vi "Sequencer.pub.vi"() -> ()   [LabVIEW 2014]
uses:
  <vilib>/Analysis/NI_AALPro.lvlib
panel:
  out "Counts":u32[](array[numeric])
  out "PMT4":u32[](array[numeric])
  out "PMT3":u32[](array[numeric])
  out "PMT2":u32[](array[numeric])
  out "PMT1":u32[](array[numeric])
  in  "Threshold":dbl=1.0
  out "CompiledSequence":string="#DopplerCooling\r\n0.9 10100000 00000000 00000000\r\n\r\n#Pump\r\n0.3 01000000 00000000 00000000\r\n\r\n#Pulsed\r\n0.2 00100000 00000000 00000000\r\n0.4 00000100 00000000 00000000\r\n0.2 00000000 10000000 00000000\r\n0.2 01000000 00000000 01000000\n"
  out "ChapterNames":string[](array[string])
  out "ChapterPositions":u32[](array[numeric])
  in  "Scan":enum32{"Time"}(tab)
  out "Now (us)":dbl=1.0 format="%.2f"
  in  "Step (us)":dbl=1.0 format="%.2f"
  in  "End (us)":dbl=1.0 format="%.2f"
  in  "Start (us)":dbl=1.0 format="%.2f"
  in  "Time Scan":bool
  in  "Chapter":u16(ring) items=["Zero", "DopplerCooling[0]", "DopplerCooling[1]", "DopplerCooling[2]", "Zero"]
  in  "Once":bool=TRUE
  in  "Sequencer Port":refnum<visa-resource-name>="COM8"
  in  "Send":bool
  out "Durations Backup":dbl[](array[numeric])
  out "Durations":dbl[](array[numeric])
  in  "Period (ns)":dbl=5.0
  out "States":string[](array[string])
  in  "Sequencer":bool
  in  "Edit":enum32{"Sequence"}(tab)
  in  "Sequence":string
  in  "Save":bool
  in  "Chapter (us)":string
  in  "Sequence File":path=path "D:/Data/Sequence/Cooling.seq"
  in  "Repeats":u32=100
  in  "Compile":bool
  in  "Data":bool
  out "Clock":string
  in  "Detect":enum32{"PMT", "TTL"}(tab)
  in  "4":bool
  in  "3":bool
  in  "2":bool
  in  "1":bool=TRUE
  in  "Save":bool
  in  "Count or State":i16(ring) items=["Count", "State"]
  in  "Fit":bool
  out "Peak":u32
  out "?":cluster{dbl[], "Axis":dbl[]}(graph)
  out "?":cluster{"Axis":dbl[], "Histogram":i32[]}(graph)
  in  "Data Chapter":i16(ring) items=["All", "DopplerCooling[2]"]
  out "Average Counts or States":dbl(graph)
  out "Average of Scans":dbl[](graph)
  out "data file":string
  out "History Data":dbl[](array[numeric])
  in  "Sweep":bool
  out "Digital Waveform Graph":digitaldata(graph)
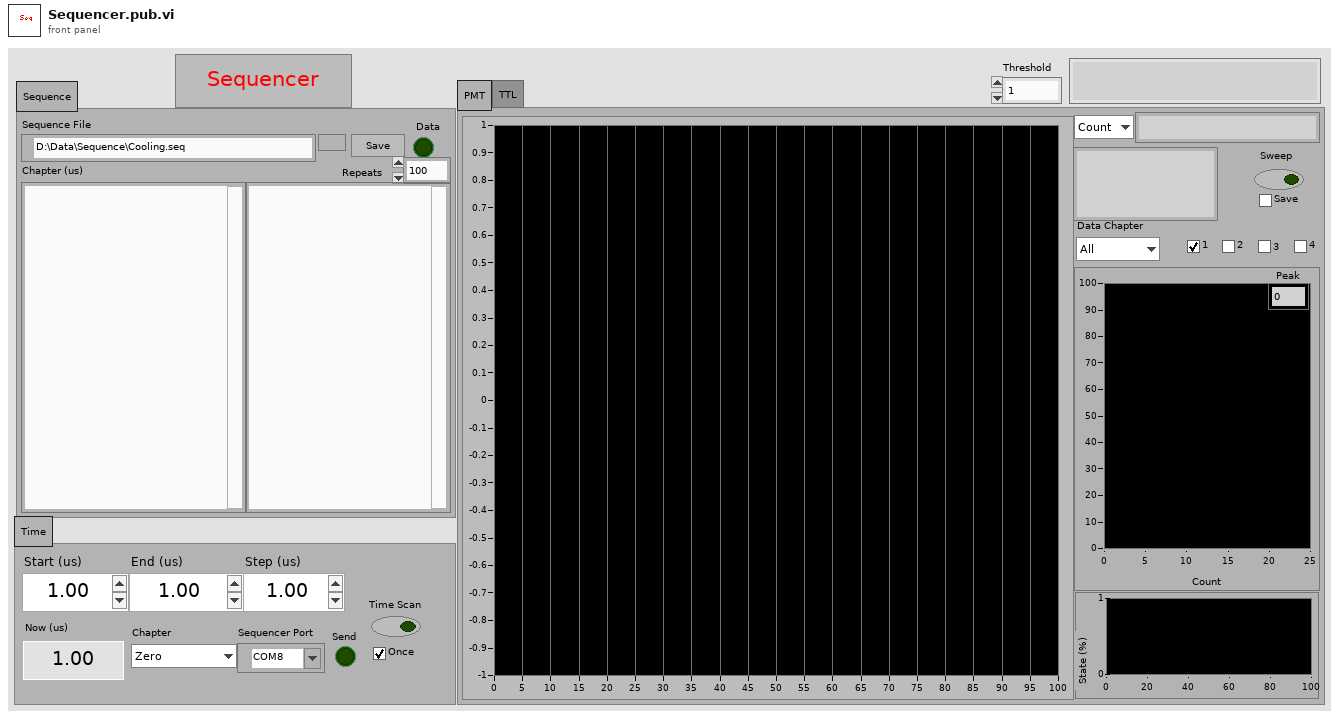
[diagram p1: front panel]
types:
  T1 = cluster{"lower":dbl, "upper":dbl, "inclusion":enum32{"lower", "upper", "both", "neither"}}[]
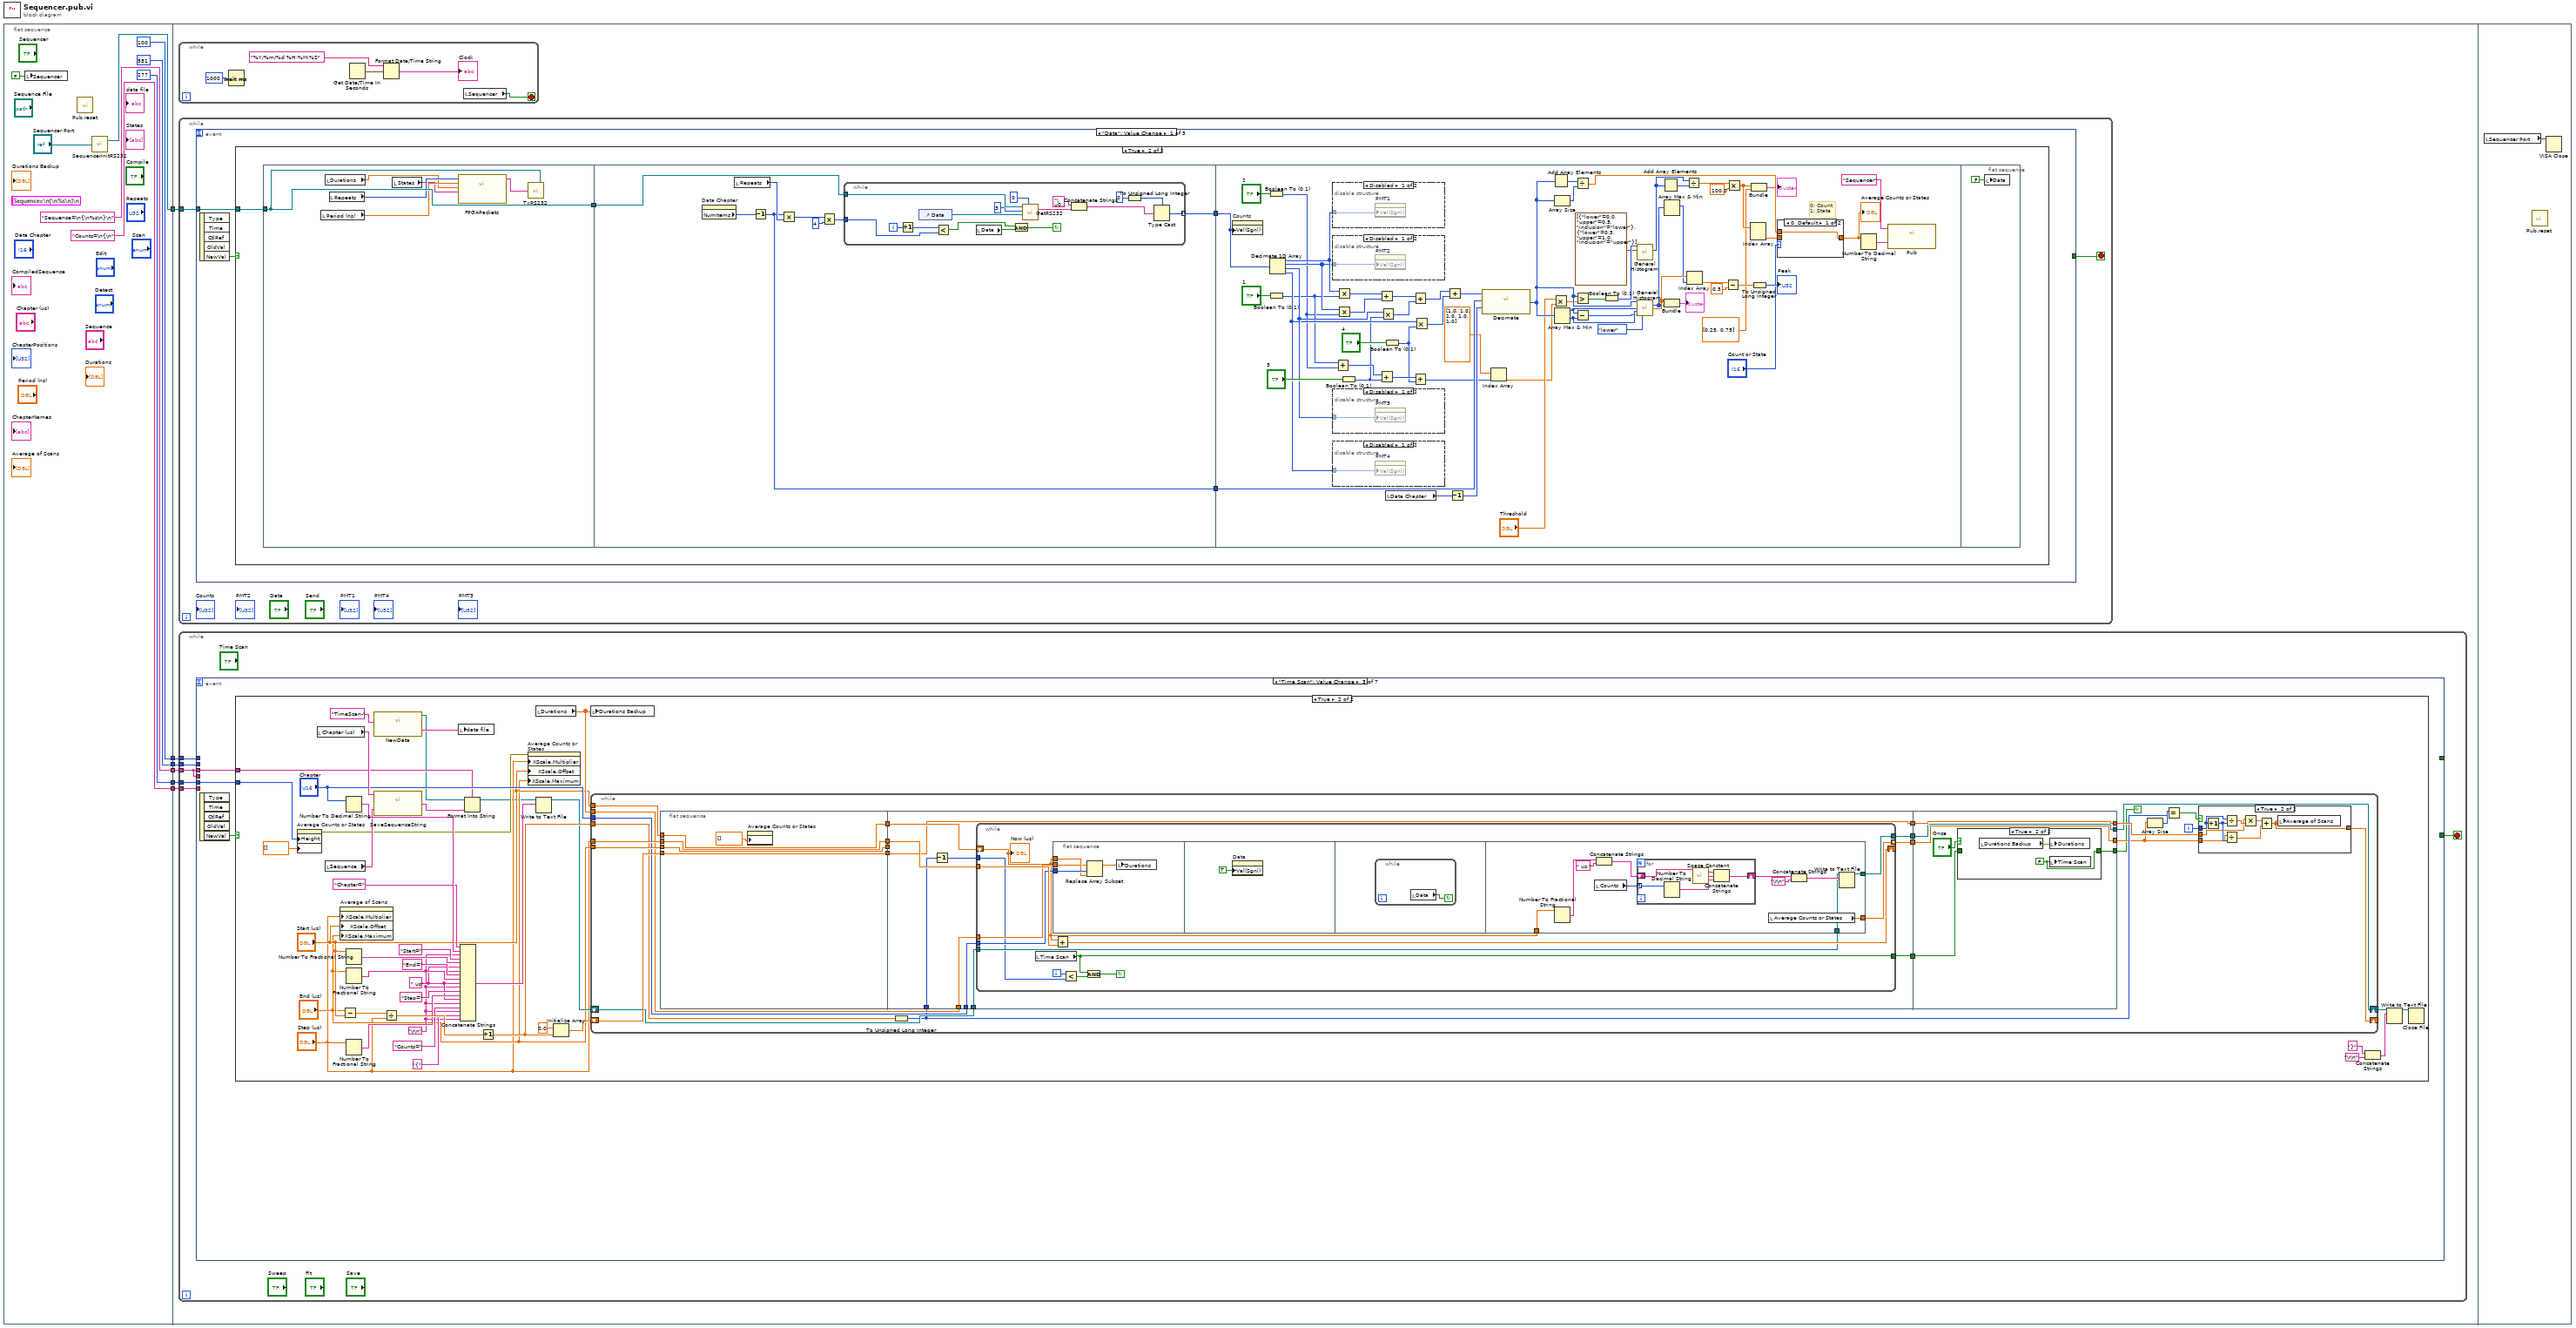
[diagram p0: block diagram]
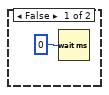
[diagram p2: hidden frame]
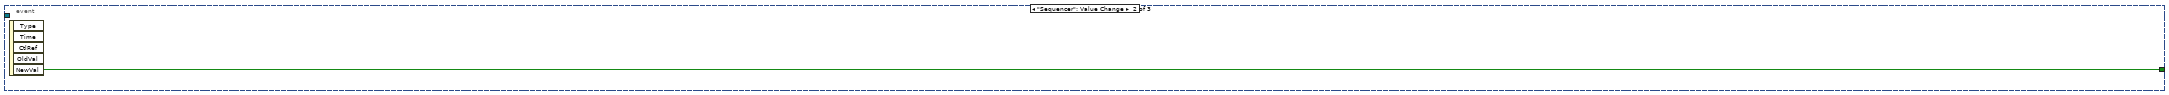
[diagram p8: hidden frame]
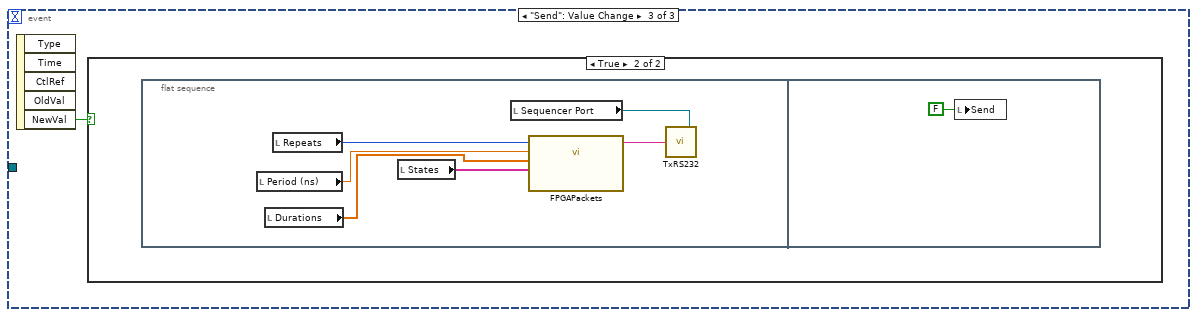
[diagram p9: hidden frame]
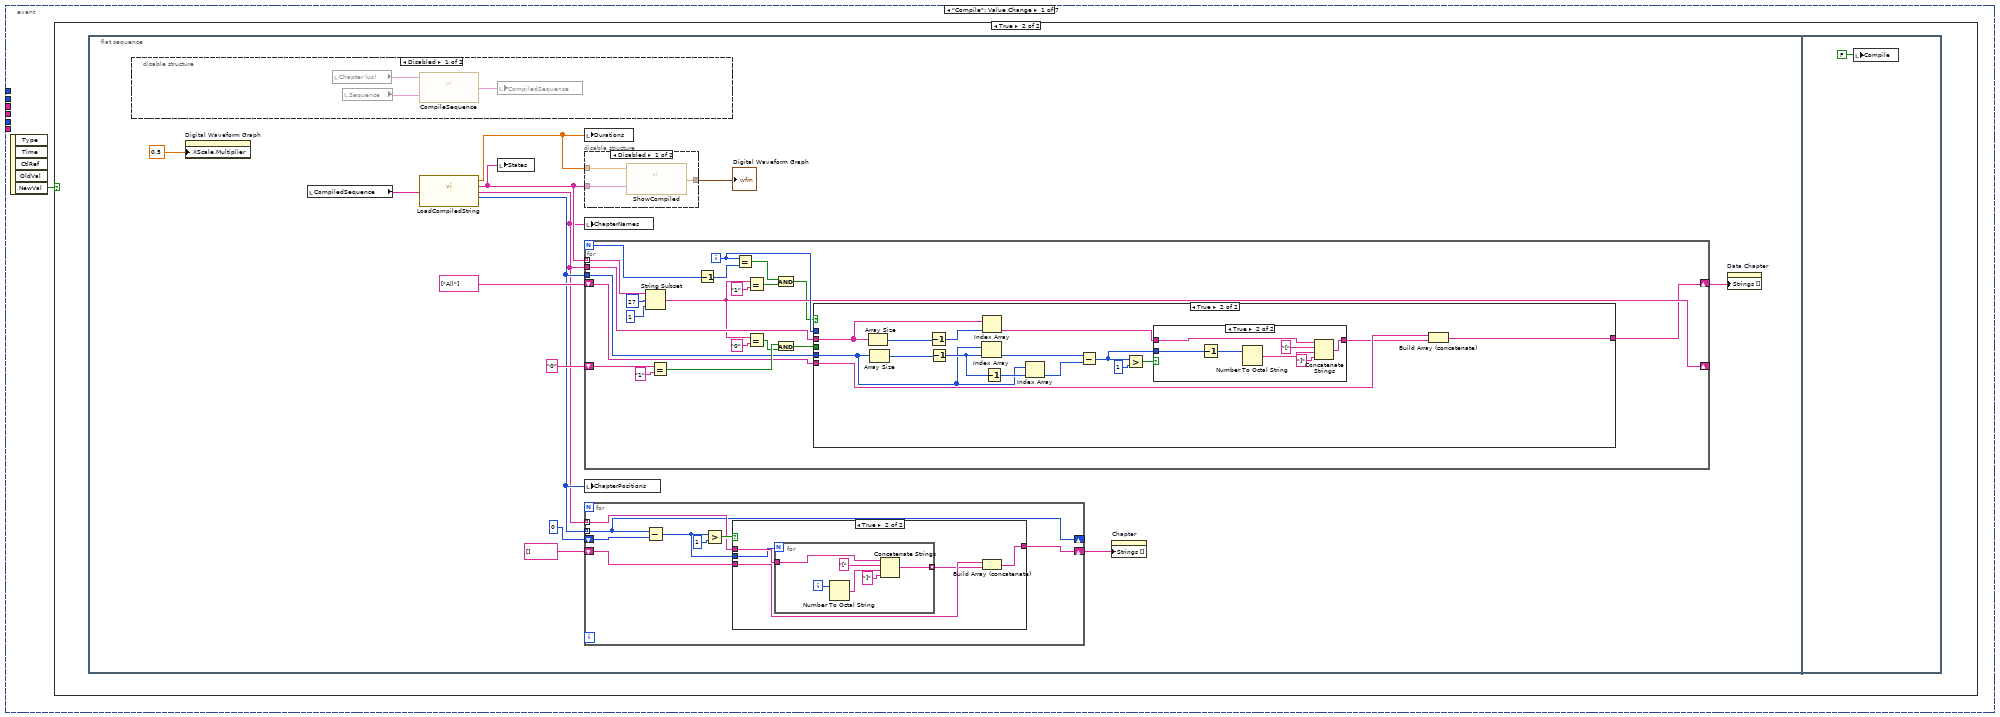
[diagram p11: hidden frame]
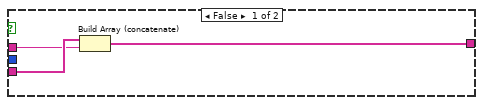
[diagram p15: hidden frame]
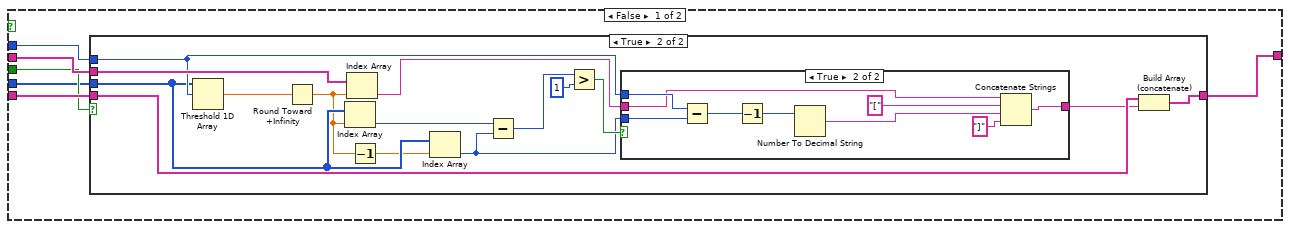
[diagram p16: hidden frame]
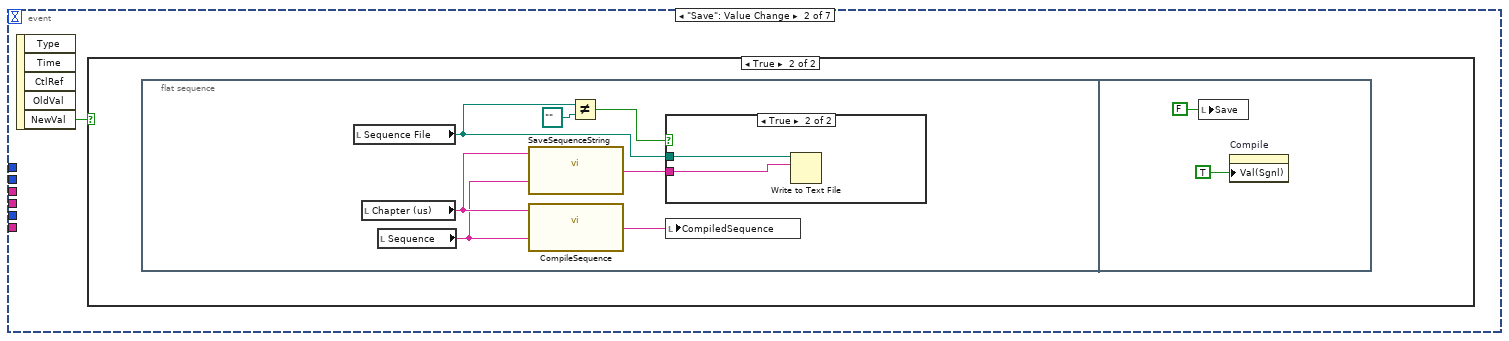
[diagram p20: hidden frame]
diagram:
  n1 = flat-sequence {
    tunnel: [w7] -> w6
    tunnel: [u32 277 ("XControl:Container Bounds:Height")] -> w5
    tunnel: [u32 551 ("Plot Area:Size:Height")] -> w4
    tunnel: [100 ("y")] -> w3
    tunnel: ["Sequence=\n{\n%s\n}\n" ("format string")] -> w2
    tunnel: ["Counts=\n{\n" ("text")] -> w1
    tunnel: w6 -> [w20]
    tunnel: w5 -> [w19]
    tunnel: w4 -> [w18]
    tunnel: w3 -> [w17]
    tunnel: w2 -> [w16]
    tunnel: w1 -> [w15]
    frame #0 {
      n2 = local write "Sequencer"(FALSE ("Sequencer")) -> ()
      n3 = call "Pub.reset.vi"() -> ()  [unwired: 12 in]
      n4 = call "SequencerInitRS232.vi"("VISA resource name"="Sequencer Port") -> ("reference out"=w7:refnum<visa-resource-name>)  [unwired: 1 out]
    }
    frame #1 {
      n5 = while {
        stop <- w21 stop-if-true
        n6 = Wait (ms)(milliseconds to wait=u32 1000) -> ()  [unwired: 1 out]
        n7 = Get Date/Time In Seconds() -> (seconds since 1Jan1904=w25:timestamp)
        n8 = Format Date/Time String(time format string (%c)="%Y/%m/%d %H:%M:%S", seconds (now)=w25) -> (date/time string=→"Clock":string)  [unwired: 1 in]
        n9 = local read "Sequencer"() -> (w21:bool)
      }
      n10 = while {
        tunnel: w20 -> [w27]
        stop <- w26 stop-if-true
        n11 = event shown="[0] \"Data\": Value Change" {
          selector: _ -> [_ _ _]
          dyn-events: _ -> [_ _ _]
          timeout: _ -> [_ _ _]
          tunnel: w27 -> [w29 _ _]
          tunnel: [_ w133 _] -> w26
          event "Data": Value Change {
            n12 = event-data() -> ("NewVal"=w28:bool)  [unwired: 1 in, 4 out]
            n13 = case shown="True" w28 {
              tunnel: w29 -> [_ w34]
              frame False {
                n14 = Wait (ms)(milliseconds to wait=u32 0) -> ()  [unwired: 1 out]
              }
              frame True {
                n15 = flat-sequence {
                  tunnel: w34 -> [w39]
                  tunnel: [w39] -> w31
                  tunnel: [w46] -> w33
                  tunnel: [w44] -> w32
                  tunnel: w31 -> [w48]
                  tunnel: w33 -> [w94]
                  tunnel: w32 -> [w100]
                  frame #0 {
                    n16 = local read "Period (ns)"() -> (w37:dbl)
                    n17 = local read "Durations"() -> (w36:dbl[])
                    n18 = local read "Repeats"() -> (w38:u32)
                    n19 = local read "States"() -> (w35:string[])
                    n20 = call "FPGAPackets.vi"("Repeats"=w38, "Period (ns)"=w37, "Durations"=w36, "States"=w35) -> ("Packets"=w40:string)  [unwired: 1 in, 1 out]
                    n21 = call "TxRS232.vi"("VISA resource name"=w39, "Data"=w40) -> ()
                  }
                  frame #1 {
                    n22 = property on="Data Chapter" class="Ring (strict)"() -> ("NumItems"=w47:u32)  [unwired: 2 in, 2 out]
                    n23 = local read "Repeats"() -> (w45:u32)
                    n24 = Decrement(x=w47) -> (x-1=w44:u32)
                    n25 = Multiply(x=w44, y=w45) -> (x*y=w43:u32)
                    n26 = Multiply(x=w43, y=u32 4) -> (x*y=w42:u32)
                    n27 = while {
                      tunnel: w48 -> [w56]
                      tunnel: [w57] -> w46 mode=indexing
                      tunnel: w42 -> [w52]
                      i -> [w51]
                      stop <- w60 continue-if-true
                      n28 = Increment(x=w51) -> (x+1=w50:i32)
                      n29 = control-ref of="Data"() -> (w53:refnum<vi>)
                      n30 = Less?(x=w50, y=w52) -> (x < y?=w59:bool)
                      n31 = local read "Data"() -> (w61:bool)
                      n32 = And(x=w59, y=w61) -> (x .and. y?=w60:bool)
                      n33 = call "GetRS232.vi"("VISA resource name"=w56, "Bytes To Read"=3, "Control"=w53, "Limit"=0) -> ("Data"=w54:string)  [unwired: 1 in, 1 out]
                      n34 = Concatenate Strings("\u0000" ("string"), w54) -> (w58:string)
                      n35 = To Unsigned Long Integer(number=u32 0) -> (unsigned 32bit integer=w64:u32)
                      n36 = Type Cast(type=w64, x=w58) -> (*(type *) &x=w57:u32)
                    }
                  }
                  frame #2 {
                    # "0: Count\n1: State"
                    n37 = property on="Counts" class="Arr (strict)"("Val(Sgnl)"=w94) -> ()  [unwired: 2 in, 2 out]
                    n38 = Boolean To (0,1)(Boolean="2") -> (0, 1=w77:i16)
                    n39 = Boolean To (0,1)(Boolean="1") -> (0, 1=w78:i16)
                    n40 = Decimate 1D Array(w94) -> (w93:u32[], w90:u32[], w86:u32[], w83:u32[])
                    n41 = disable-structure shown="Disabled" {
                      disable-tunnel: w93 -> [w129 _]
                      frame Disabled {
                        n42 = property on="PMT1" class="Arr (strict)"("Val(Sgnl)"=w129) -> ()  [unwired: 2 in, 2 out]
                      }
                      frame Enabled {
                      }
                    }
                    n43 = disable-structure shown="Disabled" {
                      disable-tunnel: w90 -> [w128 _]
                      frame Disabled {
                        n44 = property on="PMT2" class="Arr (strict)"("Val(Sgnl)"=w128) -> ()  [unwired: 2 in, 2 out]
                      }
                      frame Enabled {
                      }
                    }
                    n45 = disable-structure shown="Disabled" {
                      disable-tunnel: w86 -> [w127 _]
                      frame Disabled {
                        n46 = property on="PMT3" class="Arr (strict)"("Val(Sgnl)"=w127) -> ()  [unwired: 2 in, 2 out]
                      }
                      frame Enabled {
                      }
                    }
                    n47 = disable-structure shown="Disabled" {
                      disable-tunnel: w83 -> [w126 _]
                      frame Disabled {
                        n48 = property on="PMT4" class="Arr (strict)"("Val(Sgnl)"=w126) -> ()  [unwired: 2 in, 2 out]
                      }
                      frame Enabled {
                      }
                    }
                    n49 = Add(x=w78, y=w77) -> (x+y=w76:i16)
                    n50 = Multiply(x=w93, y=w78) -> (x*y=w79:u32[])
                    n51 = Multiply(x=w90, y=w77) -> (x*y=w89:u32[])
                    n52 = Boolean To (0,1)(Boolean="3") -> (0, 1=w75:i16)
                    n53 = Add(x=w79, y=w89) -> (x+y=w84:u32[])
                    n54 = Add(x=w76, y=w75) -> (x+y=w74:i16)
                    n55 = Multiply(x=w86, y=w75) -> (x*y=w85:u32[])
                    n56 = Boolean To (0,1)(Boolean="4") -> (0, 1=w73:i16)
                    n57 = local read "Data Chapter"() -> (w98:i16)
                    n58 = Add(x=w84, y=w85) -> (x+y=w81:u32[])
                    n59 = Add(x=w74, y=w73) -> (x+y=w68:i16)
                    n60 = Multiply(x=w83, y=w73) -> (x*y=w82:u32[])
                    n61 = Add(x=w81, y=w82) -> (x+y=w80:u32[])
                    n62 = Decrement(x=w98) -> (x-1=w97:i16)
                    n63 = call "Decimate.vi"("i"=w97, "n"=w100, "Input Array"=w80) -> ("Decimated Array"=w122:u32[])
                    n64 = Index Array(array=dbl[] [1.0, 1.0, 1.0, 1.0, 1.0], index=w68) -> (element=w70:dbl)
                    n65 = Add Array Elements(numeric array=w122) -> (sum=w121:u32)
                    n66 = Multiply(x="Threshold", y=w70) -> (x*y=w69:dbl)
                    n67 = Array Size(array=w122) -> (size(s)=w120:i32)
                    n68 = Array Max & Min(array=w122) -> (max value=w101:u32, min value=w111:u32)  [unwired: 2 out]
                    n69 = Divide(x=w121, y=w120) -> (x/y=w124:dbl)
                    n70 = Greater?(x=w122, y=w69) -> (0:w107:bool[])
                    n71 = Subtract(x=w101, y=w111) -> (x-y=w110:u32)
                    n72 = Boolean To (0,1)(Boolean=w107) -> (0, 1=w106:i16[])
                    n73 = call <vilib>:"General Histogram.vi"("X"=w106, "Bins"=T1 [{"lower"=0.0, "upper"=0.5, "inclusion"=enum."lower"}, {"lower"=0.5, "upper"=1.0, "inclusion"=enum."upper"}]) -> ("Histogram"=w104:i32[])  [unwired: 9 in, 4 out]
                    n74 = call <vilib>:"General Histogram.vi"("X"=w122, "max"=w101, "min"=w111, "# bins"=w110, "inclusion"=enum32{"lower", "upper"}."lower") -> ("Histogram"=w112:i32[], "Axis"=w114:dbl[])  [unwired: 6 in, 3 out]
                    n75 = Add Array Elements(numeric array=w104) -> (sum=w105:i32)
                    n76 = Array Max & Min(array=w112) -> (max index (indices)=w113:i32)  [unwired: 3 out]
                    n77 = Bundle("Axis"=w114, "Histogram"=w112) -> (→"?":cluster{"Axis":dbl[], "Histogram":i32[]})  [unwired: 1 in]
                    n78 = Divide(x=w104, y=w105) -> (x/y=w102:dbl[])
                    n79 = Index Array(array=w114, index=w113) -> (element=w118:dbl)
                    n80 = Subtract(x=w118, y=0.5) -> (x-y=w117:dbl)
                    n81 = Multiply(x=w102, y=100.0) -> (x*y=w123:dbl[])
                    n82 = Index Array(array=w123) -> (element #2=w125:dbl)  [unwired: 2 in, 1 out]
                    n83 = Bundle(w123, "Axis"=dbl[] [0.25, 0.75]) -> (→"?":cluster{dbl[], "Axis":dbl[]})  [unwired: 1 in]
                    n84 = To Unsigned Long Integer(number=w117) -> (unsigned 32bit integer=→"Peak":u32)
                    n85 = case shown="0, Default" "Count or State" {
                      tunnel: w124 -> [w130 _]
                      tunnel: [w130 w131] -> w67
                      tunnel: w125 -> [_ w131]
                      frame 0, Default {
                      }
                      frame 1 {
                      }
                    }
                    "Average Counts or States" <- w67
                    n86 = Number To Decimal String(number=w67) -> (decimal integer string=w66:string)  [unwired: 1 in]
                    n87 = call "Pub.vi"("Msg"=w66, "Topic"="Sequencer") -> ()  [unwired: 1 in, 1 out]
                  }
                  frame #3 {
                    n88 = local write "Data"(FALSE ("Acquisition")) -> ()
                  }
                }
              }
            }
          }
          event "Sequencer": Value Change {
            n89 = event-data() -> ("NewVal"=w133:bool)  [unwired: 1 in, 4 out]
          }
          event "Send": Value Change {
            n90 = event-data() -> ("NewVal"=w134:bool)  [unwired: 1 in, 4 out]
            n91 = case shown="True" w134 {
              frame False {
              }
              frame True {
                n92 = flat-sequence {
                  frame #0 {
                    n93 = local read "Period (ns)"() -> (w138:dbl)
                    n94 = local read "Durations"() -> (w136:dbl[])
                    n95 = local read "Repeats"() -> (w137:u32)
                    n96 = local read "States"() -> (w139:string[])
                    n97 = local read "Sequencer Port"() -> (w140:refnum<visa-resource-name>)
                    n98 = call "FPGAPackets.vi"("Repeats"=w137, "Period (ns)"=w138, "Durations"=w136, "States"=w139) -> ("Packets"=w135:string)  [unwired: 1 in, 1 out]
                    n99 = call "TxRS232.vi"("VISA resource name"=w140, "Data"=w135) -> ()
                  }
                  frame #1 {
                    n100 = local write "Send"(FALSE ("Send")) -> ()
                  }
                }
              }
            }
          }
        }
      }
      n101 = while {
        tunnel: w19 -> [w146]
        tunnel: w18 -> [w145]
        tunnel: w17 -> [w144]
        tunnel: w16 -> [w142]
        tunnel: w15 -> [w143]
        stop <- w147 stop-if-true
        n102 = event shown="[2] \"Time Scan\": Value Change" {
          selector: _ -> [_ _ _ _ _ _ _]
          dyn-events: _ -> [_ _ _ _ _ _ _]
          timeout: _ -> [_ _ _ _ _ _ _]
          tunnel: [_ _ _ _ _ _ w497] -> _
          tunnel: [_ _ _ _ _ _ w497] -> w147
          tunnel: w146 -> [_ _ w281 _ _ _ _]
          tunnel: w145 -> [_ _ _ _ _ w434 _]
          tunnel: w144 -> [_ _ _ _ _ w433 _]
          tunnel: w142 -> [_ _ _ _ _ w432 _]
          tunnel: w143 -> [_ _ _ _ _ w431 _]
          tunnel: w142 -> [_ _ w280 _ _ _ _]
          event "Compile": Value Change {
            n103 = event-data() -> ("NewVal"=w148:bool)  [unwired: 1 in, 4 out]
            n104 = case shown="True" w148 {
              frame False {
              }
              frame True {
                n105 = flat-sequence {
                  frame #0 {
                    n106 = disable-structure shown="Disabled" {
                      frame Disabled {
                        n107 = local read "Chapter (us)"() -> (w167:string)
                        n108 = local read "Sequence"() -> (w166:string)
                        n109 = call "CompileSequence.vi"("Sequence"=w166, "Chapter"=w167) -> ("Compiled Sequence"=w165:string)
                        n110 = local write "CompiledSequence"(w165) -> ()
                      }
                      frame Enabled {
                      }
                    }
                    n111 = property on="Digital Waveform Graph" class="DigitalGraph (strict)"("XScale.Multiplier"=0.5 ("X Scale.Offset and Multiplier:Multiplier")) -> ()  [unwired: 2 in, 2 out]
                    n112 = local read "CompiledSequence"() -> (w149:string)
                    n113 = call "LoadCompiledString.vi"("Compiled String"=w149) -> ("Durations"=w160:dbl[], "States"=w159:string[], "ChapterNames"=w150:string[], "ChapterPositions"=w151:u32[])
                    n114 = local write "States"(w159) -> ()
                    n115 = local write "Durations"(w160) -> ()
                    n116 = disable-structure shown="Disabled" {
                      disable-tunnel: [w164 _] -> w161
                      disable-tunnel: w160 -> [w163 _]
                      disable-tunnel: w159 -> [w162 _]
                      frame Disabled {
                        n117 = call "ShowCompiled.vi"("States"=w162, "Durations"=w163) -> ("Digital Waveform Graph"=w164:digitaldata)
                      }
                      frame Enabled {
                      }
                    }
                    "Digital Waveform Graph" <- w161
                    n118 = local write "ChapterNames"(w150) -> ()
                    n119 = for {
                      N -> [w201]
                      tunnel: w159 -> [w210] mode=indexing
                      shift-right: [w198] -> _
                      shift-left: "0" -> [w208]
                      tunnel: w150 -> [w204]
                      shift-right: [w193] -> w154
                      shift-left: string[] ["All"] -> [w192]
                      tunnel: w151 -> [w191]
                      i -> [w202]
                      n120 = String Subset(string=w210, offset (0)=27, length (rest)=1 ("length (rest)")) -> (substring=w198:string)
                      n121 = Equal?(x=w208, y="1") -> (x = y?=w206:bool)
                      n122 = Decrement(x=w201) -> (x-1=w200:i32)
                      n123 = Equal?(x=w202, y=w200) -> (x = y?=w197:bool)
                      n124 = Equal?(x=w198, y="1") -> (x = y?=w196:bool)
                      n125 = Equal?(x=w198, y="0") -> (x = y?=w203:bool)
                      n126 = And(x=w197, y=w196) -> (x .and. y?=w195:bool)
                      n127 = And(x=w206, y=w203) -> (x .and. y?=w194:bool)
                      n128 = case shown="True" w195 {
                        tunnel: w204 -> [w216 w256]
                        tunnel: w192 -> [w215 w258]
                        tunnel: w202 -> [w214 _]
                        tunnel: w194 -> [w213 _]
                        tunnel: [w212 w257] -> w193
                        tunnel: w191 -> [w211 w250]
                        frame False {
                          n129 = case shown="True" w213 {
                            tunnel: w214 -> [_ w228]
                            tunnel: w216 -> [_ w229]
                            tunnel: w215 -> [w217 w231]
                            tunnel: [w217 w232] -> w212
                            tunnel: w211 -> [_ w225]
                            frame False {
                            }
                            frame True {
                              n130 = Threshold 1D Array(2:w228, 3:w225) -> (0:w230:dbl)  [unwired: 1 in]
                              n131 = Round Toward +Infinity(x=w230) -> (ceil(x): smallest int >= x=w223:dbl)
                              n132 = Index Array(array=w225, index=w223) -> (element=w222:u32)
                              n133 = Index Array(array=w229, index=w223) -> (element=w226:string)
                              n134 = Decrement(x=w223) -> (x-1=w224:dbl)
                              n135 = Index Array(array=w225, index=w224) -> (element=w218:u32)
                              n136 = Subtract(x=w222, y=w218) -> (x-y=w221:u32)
                              n137 = Greater?(x=w221, y=u32 1) -> (0:w219:bool)
                              n138 = case shown="True" w219 {
                                tunnel: w228 -> [_ w242]
                                tunnel: [w233 w236] -> w227
                                tunnel: w226 -> [w233 w235]
                                tunnel: w218 -> [_ w234]
                                frame False {
                                }
                                frame True {
                                n139 = Subtract(x=w242, y=w234) -> (x-y=w241:u32)
                                n140 = Decrement(x=w241) -> (x-1=w240:u32)
                                n141 = Number To Decimal String(number=w240) -> (decimal integer string=w237:string)  [unwired: 1 in]
                                n142 = Concatenate Strings(w235, "[" ("element"), w237, "]" ("element")) -> (w236:string)
                                }
                              }
                              n143 = Build Array (concatenate)(w231, w227) -> (w232:string[])
                            }
                          }
                        }
                        frame True {
                          n144 = Array Size(array=w256) -> (size(s)=w255:i32)
                          n145 = Array Size(array=w250) -> (size(s)=w253:i32)
                          n146 = Decrement(x=w255) -> (x-1=w254:i32)
                          n147 = Decrement(x=w253) -> (x-1=w252:i32)
                          n148 = Index Array(array=w250, index=w252) -> (element=w249:u32)
                          n149 = Index Array(array=w256, index=w254) -> (element=w245:string)
                          n150 = Decrement(x=w252) -> (x-1=w251:i32)
                          n151 = Index Array(array=w250, index=w251) -> (element=w248:u32)
                          n152 = Subtract(x=w249, y=w248) -> (x-y=w243:u32)
                          n153 = Greater?(x=w243, y=u32 1) -> (0:w246:bool)
                          n154 = case shown="True" w246 {
                            tunnel: w245 -> [w259 w266]
                            tunnel: [w259 w260] -> w244
                            tunnel: w243 -> [_ w263]
                            frame False {
                            }
                            frame True {
                              n155 = Decrement(x=w263) -> (x-1=w262:u32)
                              n156 = Number To Octal String(2:w262) -> (0:w261:string)  [unwired: 1 in]
                              n157 = Concatenate Strings(w266, "[" ("string"), w261, "]" ("string")) -> (w260:string)
                            }
                          }
                          n158 = Build Array (concatenate)(w258, w244) -> (w257:string[])
                        }
                      }
                    }
                    n159 = local write "ChapterPositions"(w151) -> ()
                    n160 = for {
                      tunnel: w151 -> [w168] mode=indexing
                      tunnel: w150 -> [w169] mode=indexing
                      shift-right: [w168] -> _
                      shift-left: u32 0 ("initial scan location") -> [w175]
                      shift-right: [w170] -> w156
                      shift-left: string[] [] -> [w171]
                      n161 = Subtract(x=w168, y=w175) -> (x-y=w172:u32)
                      n162 = Greater?(x=w172, y=u32 1) -> (0:w174:bool)
                      n163 = case shown="True" w174 {
                        tunnel: w169 -> [w177 w183]
                        tunnel: w172 -> [_ w182]
                        tunnel: w171 -> [w178 w181]
                        tunnel: [w176 w179] -> w170
                        frame False {
                          n164 = Build Array (concatenate)(w178, w177) -> (w176:string[])
                        }
                        frame True {
                          n165 = for {
                            N: w182 -> [_]
                            tunnel: w183 -> [w188]
                            tunnel: [w187] -> w180 mode=indexing
                            i -> [w189]
                            n166 = Number To Octal String(2:w189) -> (0:w186:string)  [unwired: 1 in]
                            n167 = Concatenate Strings(w188, "[" ("string"), w186, "]" ("string")) -> (w187:string)
                          }
                          n168 = Build Array (concatenate)(w181, w180) -> (w179:string[])
                        }
                      }
                    }
                    n169 = property on="Chapter" class="Ring (strict)"("Strings []"=w156) -> ()  [unwired: 2 in, 2 out]
                    n170 = property on="Data Chapter" class="Ring (strict)"("Strings []"=w154) -> ()  [unwired: 2 in, 2 out]
                  }
                  frame #1 {
                    n171 = local write "Compile"(FALSE ("Compile")) -> ()
                  }
                }
              }
            }
          }
          event "Save": Value Change {
            n172 = event-data() -> ("NewVal"=w268:bool)  [unwired: 1 in, 4 out]
            n173 = case shown="True" w268 {
              frame False {
              }
              frame True {
                n174 = flat-sequence {
                  frame #0 {
                    n175 = local read "Sequence File"() -> (w273:path)
                    n176 = local read "Chapter (us)"() -> (w271:string)
                    n177 = local read "Sequence"() -> (w270:string)
                    n178 = call "SaveSequenceString.vi"("Sequence"=w270, "Chapter"=w271) -> ("Sequence String"=w272:string)
                    n179 = call "CompileSequence.vi"("Sequence"=w270, "Chapter"=w271) -> ("Compiled Sequence"=w269:string)
                    n180 = Not Equal?(x=w273, y=path "") -> (x != y?=w275:bool)
                    n181 = case shown="True" w275 {
                      tunnel: w273 -> [_ w277]
                      tunnel: w272 -> [_ w276]
                      frame False {
                      }
                      frame True {
                        n182 = Write to Text File(file (use dialog)=w277, text=w276) -> ()  [unwired: 2 in, 3 out]
                      }
                    }
                    n183 = local write "CompiledSequence"(w269) -> ()
                  }
                  frame #1 {
                    n184 = local write "Save"(FALSE ("Compile")) -> ()
                    n185 = property on="Compile" class="Bool (strict)"("Val(Sgnl)"=TRUE ("Value (Signaling)")) -> ()  [unwired: 2 in, 2 out]
                  }
                }
              }
            }
          }
          event "Time Scan": Value Change {
            n186 = event-data() -> ("NewVal"=w282:bool)  [unwired: 1 in, 4 out]
            n187 = case shown="True" w282 {
              tunnel: w281 -> [_ w294]
              tunnel: w280 -> [_ w287]
              frame False {
                n188 = local read "Durations Backup"() -> (w283:dbl[])
                n189 = local write "Durations"(w283) -> ()
              }
              frame True {
                w307 = " us" ("string")
                w304 = "\r\n"
                n190 = property on="Average Counts or States" class="WFChart (strict)"("Height"=w294, "History Data"=dbl[] []) -> (error out=w293:errorcluster)  [unwired: 2 in, 1 out]
                n191 = local read "Chapter (us)"() -> (w314:string)
                n192 = local read "Sequence"() -> (w315:string)
                n193 = property on="Average of Scans" class="WFGraph (strict)"("XScale.Multiplier"="Step (us)", "XScale.Offset"="Start (us)", "XScale.Maximum"="End (us)") -> ()  [unwired: 2 in, 2 out]
                n194 = Subtract(x="End (us)", y="Start (us)") -> (x-y=w322:dbl)
                n195 = Number To Decimal String(number="Chapter") -> (decimal integer string=w318:string)  [unwired: 1 in]
                n196 = Number To Fractional String(number="Start (us)") -> (F-format string=w312:string)  [unwired: 3 in]
                n197 = Number To Fractional String(number="End (us)") -> (F-format string=w310:string)  [unwired: 3 in]
                n198 = Number To Fractional String(number="Step (us)") -> (F-format string=w308:string)  [unwired: 3 in]
                n199 = call "NewData.vi"("Prefix"="TimeScan-" ("string")) -> ("data file name"=w291:string, "data file refnum"=w285:refnum<file>)  [unwired: 2 in]
                n200 = call "SaveSequenceString.vi"("Sequence"=w315, "Chapter"=w314) -> ("Sequence String"=w286:string)
                n201 = Divide(x=w322, y="Step (us)") -> (x/y=w321:dbl)
                n202 = local write "data file"(w291) -> ()
                n203 = Concatenate Strings("Chapter=" ("string"), w318, w304, "Start=" ("string"), w312, w307, w304, "End=" ("string"), w310, w307, w304, "Step=" ("string"), w308, w307, w304, "Counts=" ("string"), w304, "{" ("string"), w304) -> (w316:string)
                n204 = Format Into String(format string=w287, initial string=w285, w286) -> (resulting string=w284:refnum<file>)  [unwired: 1 in, 1 out]
                n205 = Increment(x=w321) -> (x+1=w320:dbl)
                n206 = property on="Average Counts or States" class="WFChart (strict)"(error in=w293, "XScale.Multiplier"="Step (us)", "XScale.Offset"="Start (us)", "XScale.Maximum"="End (us)") -> ()  [unwired: 1 in, 2 out]
                n207 = local read "Durations"() -> (w297:dbl[])
                n208 = Write to Text File(file (use dialog)=w284, text=w316) -> (refnum out=w303:refnum<file>)  [unwired: 2 in, 2 out]
                n209 = Initialize Array(0.0 ("element"), w320) -> (w296:dbl[])
                n210 = local write "Durations Backup"(w297) -> ()
                n211 = while {
                  tunnel: "Start (us)" -> [w348]
                  tunnel: "Step (us)" -> [w347]
                  tunnel: "End (us)" -> [w346]
                  shift-right: [w336] -> _
                  shift-left: w296 -> [w345]
                  tunnel: w320 -> [w332]
                  tunnel: "Chapter" -> [w335]
                  shift-right: [w334] -> w301
                  shift-left: w303 -> [w333]
                  tunnel: w297 -> [w331]
                  i -> [w338]
                  stop <- w324 continue-if-true
                  n212 = flat-sequence {
                    tunnel: w345 -> [w359]
                    tunnel: w346 -> [w360]
                    tunnel: w347 -> [w361]
                    tunnel: w348 -> [w362]
                    tunnel: [w362] -> w344
                    tunnel: [w361] -> w343
                    tunnel: [w360] -> w342
                    tunnel: [w359] -> w341
                    tunnel: w344 -> [w373]
                    tunnel: w343 -> [w372]
                    tunnel: w342 -> [_]
                    tunnel: w341 -> [w371]
                    tunnel: w335 -> [w369]
                    tunnel: w333 -> [w368]
                    tunnel: w331 -> [w366]
                    tunnel: w330 -> [w365]
                    tunnel: [w371] -> w328
                    tunnel: [w370] -> w327
                    tunnel: [w367] -> w326
                    tunnel: [w363] -> w325
                    tunnel: [w412] -> w329
                    tunnel: [w413] -> w334
                    tunnel: [w409] -> w324
                    tunnel: [w414] -> w337
                    tunnel: w328 -> [w414]
                    tunnel: w327 -> [w410]
                    tunnel: w326 -> [w413]
                    tunnel: w325 -> [w412]
                    frame #0 {
                      n213 = property on="Average Counts or States" class="WFChart (strict)"("History Data"=dbl[] []) -> ()  [unwired: 2 in, 2 out]
                    }
                    frame #1 {
                      n214 = Decrement(x=w365) -> (x-1=w364:u32)
                      n215 = while {
                        shift-right: [w386] -> _
                        shift-left: w373 -> [w374]
                        tunnel: w372 -> [w384]
                        tunnel: [w383] -> w370
                        tunnel: w369 -> [w380]
                        tunnel: w368 -> [w381]
                        tunnel: [w382] -> w367
                        tunnel: w366 -> [w379]
                        tunnel: w364 -> [w376]
                        tunnel: [w375] -> w363 mode=indexing
                        i -> [w378]
                        stop <- w385 continue-if-true
                        n216 = local read "Time Scan"() -> (w383:bool)
                        n217 = flat-sequence {
                          tunnel: w380 -> [w390]
                          tunnel: w374 -> [w389]
                          tunnel: w379 -> [w387]
                          tunnel: w374 -> [w401]
                          tunnel: w381 -> [w396]
                          tunnel: [w395] -> w382
                          tunnel: [w393] -> w375
                          frame #0 {
                            n218 = Replace Array Subset(array=w387, new element=w389, index=w390) -> (w388:dbl[])
                            n219 = local write "Durations"(w388) -> ()
                          }
                          frame #1 {
                            n220 = property on="Data" class="Bool (strict)"("Val(Sgnl)"=TRUE ("Acquisition")) -> ()  [unwired: 2 in, 2 out]
                          }
                          frame #2 {
                            n221 = while {
                              stop <- w392 continue-if-true
                              n222 = local read "Data"() -> (w392:bool)
                            }
                          }
                          frame #3 {
                            n223 = Number To Fractional String(number=w401) -> (F-format string=w403:string)  [unwired: 3 in]
                            n224 = local read "Counts"() -> (w394:u32[])
                            n225 = Concatenate Strings(w403, " us," ("string")) -> (w400:string)
                            n226 = for {
                              tunnel: w394 -> [w408] mode=indexing
                              shift-right: [w406] -> w397
                              shift-left: w400 -> [w405]
                              n227 = Number To Decimal String(number=w408) -> (decimal integer string=w407:string)  [unwired: 1 in]
                              n228 = call <vilib>:"Space Constant.vi"() -> ("String"=w404:string)
                              n229 = Concatenate Strings(w405, w404, w407) -> (w406:string)
                            }
                            n230 = local read "Average Counts or States"() -> (w393:dbl)
                            n231 = Concatenate Strings(w397, "\r\n") -> (w398:string)
                            n232 = Write to Text File(file (use dialog)=w396, text=w398) -> (refnum out=w395:refnum<file>)  [unwired: 2 in, 2 out]
                          }
                        }
                        n233 = Add(x=w374, y=w384) -> (x+y=w386:dbl)
                        n234 = Less?(x=w378, y=w376) -> (x < y?=w377:bool)
                        n235 = And(x=w383, y=w377) -> (x .and. y?=w385:bool)
                        "Now (us)" <- w374
                      }
                    }
                    frame #2 {
                      n236 = case shown="True" "Once" {
                        tunnel: w410 -> [w415 _]
                        tunnel: [w415 w417] -> w409
                        frame False {
                        }
                        frame True {
                          w417 = FALSE ("Time Scan")
                          n237 = local read "Durations Backup"() -> (w416:dbl[])
                          n238 = local write "Durations"(w416) -> ()
                          n239 = local write "Time Scan"(w417) -> ()
                        }
                      }
                    }
                  }
                  n240 = To Unsigned Long Integer(number=w332) -> (unsigned 32bit integer=w330:u32)
                  n241 = Array Size(array=w329) -> (size(s)=w339:i32)
                  n242 = Equal?(x=w339, y=w330) -> (x = y?=w340:bool)
                  n243 = case shown="True" w340 {
                    tunnel: w338 -> [_ w353]
                    tunnel: w329 -> [_ w352]
                    tunnel: w337 -> [w349 w351]
                    tunnel: [w349 w350] -> w336
                    frame False {
                    }
                    frame True {
                      n244 = Increment(x=w353) -> (x+1=w356:i32)
                      n245 = Divide(x=w353, y=w356) -> (x/y=w354:dbl)
                      n246 = Divide(x=w352, y=w356) -> (x/y=w357:dbl[])
                      n247 = Multiply(x=w351, y=w354) -> (x*y=w355:dbl[])
                      n248 = Add(x=w355, y=w357) -> (x+y=w350:dbl[])
                      n249 = local write "Average of Scans"(w350) -> ()
                    }
                  }
                }
                n250 = Concatenate Strings("}" ("string"), "\r\n") -> (w298:string)
                n251 = Write to Text File(file (use dialog)=w301, text=w298) -> (refnum out=w302:refnum<file>)  [unwired: 2 in, 2 out]
                n252 = Close File(refnum=w302) -> ()  [unwired: 1 in, 2 out]
              }
            }
          }
          event "Fit": Value Change {
            n253 = event-data() -> ("NewVal"=w418:bool)  [unwired: 1 in, 4 out]
            n254 = case shown="True" w418 {
              frame False {
              }
              frame True {
                n255 = local write "Fit"(FALSE ("Fit")) -> ()
                n256 = property on="Average Counts or States" class="WFChart (strict)"() -> ("History Data"=→"History Data":dbl[])  [unwired: 2 in, 2 out]
              }
            }
          }
          event "Sequence File": Value Change {
            n257 = event-data() -> ("NewVal"=w422:path)  [unwired: 1 in, 4 out]
            n258 = call <vilib>:"Check if File or Folder Exists.vi"("path"=w422) -> ("file or folder exists?"=w423:bool, "dup path"=w421:path)  [unwired: 8 in, 1 out]
            n259 = case shown="True" w423 {
              tunnel: w421 -> [_ w424]
              frame False {
              }
              frame True {
                n260 = flat-sequence {
                  tunnel: w424 -> [w428]
                  frame #0 {
                    n261 = Read from Text File(file (use dialog)=w428) -> (text=w429:string)  [unwired: 3 in, 3 out]
                    n262 = call "LoadSequenceString.vi"("Sequence String"=w429) -> ("Chapter"=w427:string, "Sequence"=w426:string)
                    n263 = local write "Chapter (us)"(w427) -> ()
                    n264 = call "CompileSequence.vi"("Sequence"=w426, "Chapter"=w427) -> ("Compiled Sequence"=w425:string)
                    n265 = local write "Sequence"(w426) -> ()
                    n266 = local write "CompiledSequence"(w425) -> ()
                  }
                  frame #1 {
                    n267 = property on="Compile" class="Bool (strict)"("Val(Sgnl)"=TRUE ("Value (Signaling)")) -> ()  [unwired: 2 in, 2 out]
                  }
                }
              }
            }
          }
          event "Sweep": Value Change {
            n268 = event-data() -> ("NewVal"=w435:bool)  [unwired: 1 in, 4 out]
            n269 = case shown="True" w435 {
              tunnel: w434 -> [_ w440]
              tunnel: w433 -> [_ _]
              tunnel: w432 -> [_ w439]
              tunnel: w431 -> [_ w438]
              frame False {
              }
              frame True {
                n270 = flat-sequence {
                  tunnel: w440 -> [w450]
                  tunnel: w439 -> [w445]
                  tunnel: w438 -> [w444]
                  tunnel: [w443] -> w437
                  tunnel: ["Save"] -> w436
                  tunnel: w437 -> [w467]
                  tunnel: w436 -> [w465]
                  frame #0 {
                    w451 = dbl[] [] ("History Data")
                    w448 = 0.0 ("X Scale.Offset and Multiplier:Offset")
                    w449 = 1.0 ("X Scale.Offset and Multiplier:Multiplier")
                    n271 = property on="Average Counts or States" class="WFChart (strict)"("History Data"=w451, "Height"=w450) -> (error out=w446:errorcluster)  [unwired: 2 in, 1 out]
                    n272 = property on="Average of Scans" class="WFGraph (strict)"("XScale.Multiplier"=w449, "XScale.Offset"=w448, "XScale.Maximum"=0.0 ("X Scale.Range:Maximum"), "Value"=w451) -> ()  [unwired: 2 in, 2 out]
                    n273 = case shown="True" "Save" {
                      tunnel: ["" w462] -> w442
                      tunnel: w445 -> [_ w459]
                      tunnel: w444 -> [_ w456]
                      tunnel: [_ w455] -> w443
                      frame False {
                      }
                      frame True {
                        n274 = local read "Chapter (us)"() -> (w461:string)
                        n275 = local read "Sequence"() -> (w457:string)
                        n276 = call "NewData.vi"("Prefix"="Sweep-") -> ("data file name"=w462:string, "data file refnum"=w460:refnum<file>)  [unwired: 2 in]
                        n277 = call "SaveSequenceString.vi"("Sequence"=w457, "Chapter"=w461) -> ("Sequence String"=w458:string)
                        n278 = Format Into String(format string=w459, initial string=w460, w458) -> (resulting string=w454:refnum<file>)  [unwired: 1 in, 1 out]
                        n279 = Write to Text File(file (use dialog)=w454, text=w456) -> (refnum out=w455:refnum<file>)  [unwired: 2 in, 2 out]
                      }
                    }
                    n280 = property on="Average Counts or States" class="WFChart (strict)"(error in=w446, "XScale.Multiplier"=w449, "XScale.Offset"=w448, "XScale.Maximum"=100.0 ("X Scale.Range:Maximum")) -> ()  [unwired: 1 in, 2 out]
                    n281 = local write "data file"(w442) -> ()
                  }
                  frame #1 {
                    n282 = while {
                      tunnel: [w474] -> w466
                      tunnel: w467 -> [w473]
                      tunnel: w465 -> [w472]
                      tunnel: [w472] -> w464
                      i -> [w471]
                      stop <- w475 continue-if-true
                      n283 = flat-sequence {
                        tunnel: [w481] -> w474
                        tunnel: w473 -> [w480]
                        tunnel: w472 -> [w479]
                        tunnel: w471 -> [w478]
                        frame #0 {
                          n284 = property on="Data" class="Bool (strict)"("Val(Sgnl)"=TRUE ("Value (Signaling)")) -> ()  [unwired: 2 in, 2 out]
                        }
                        frame #1 {
                          n285 = while {
                            stop <- w477 continue-if-true
                            n286 = local read "Data"() -> (w477:bool)
                          }
                        }
                        frame #2 {
                          n287 = case shown="True" w479 {
                            tunnel: [w482 w487] -> w481
                            tunnel: w480 -> [w482 w486]
                            tunnel: w478 -> [_ w483]
                            frame False {
                            }
                            frame True {
                              n288 = local read "Counts"() -> (w491:u32[])
                              n289 = Format Into String(format string="%d One,", w483) -> (resulting string=w484:string)  [unwired: 2 in, 1 out]
                              n290 = for {
                                tunnel: w491 -> [w496] mode=indexing
                                shift-right: [w494] -> w490
                                shift-left: w484 -> [w493]
                                n291 = Number To Decimal String(number=w496) -> (decimal integer string=w495:string)  [unwired: 1 in]
                                n292 = call <vilib>:"Space Constant.vi"() -> ("String"=w492:string)
                                n293 = Concatenate Strings(w493, w492, w495) -> (w494:string)
                              }
                              n294 = Concatenate Strings(w490, "\r\n") -> (w488:string)
                              n295 = Write to Text File(file (use dialog)=w486, text=w488) -> (refnum out=w487:refnum<file>)  [unwired: 2 in, 2 out]
                            }
                          }
                        }
                      }
                      n296 = local read "Sweep"() -> (w475:bool)
                    }
                    n297 = case shown="True" w464 {
                      tunnel: w466 -> [_ w469]
                      frame False {
                      }
                      frame True {
                        n298 = Write to Text File(file (use dialog)=w469, text="}\n") -> (refnum out=w470:refnum<file>)  [unwired: 2 in, 2 out]
                        n299 = Close File(refnum=w470) -> ()  [unwired: 1 in, 2 out]
                      }
                    }
                  }
                }
              }
            }
          }
          event "Sequencer": Value Change {
            n300 = event-data() -> ("NewVal"=w497:bool)  [unwired: 1 in, 4 out]
          }
        }
      }
    }
    frame #2 {
      n301 = local read "Sequencer Port"() -> (w498:refnum<visa-resource-name>)
      n302 = call "Pub.reset.vi"() -> ()  [unwired: 12 in]
      n303 = VISA Close(VISA resource name=w498) -> ()  [unwired: 1 in, 1 out]
    }
  }
